vi "Get_parts_list.vi"(7 "LabVIEW Web Service Request":refnum<class "Web Request.lvclass">) -> (2 "Parts_list":cluster{"String":string, "Value":string}[](array[cluster])=[{"String"="Пластина", "Value"="plate.png"}, {"String"="Вал", "Value"="shaft.png"}, {"String"="Ось", "Value"="axis.png"}, {"String"="Диск", "Value"="disk.png"}, {"String"="Кольцо", "Value"="ring.png"}, {"String"="Втулка", "Value"="bushing.png"}, {"String"="Крыльчатка", "Value"="impeller.png"}, {"String"="Лезвийный инструмент", "Value"="blade_tool.png"}])   [LabVIEW 2020]
uses:
  <vilib>/wsapi/Web Request.lvclass
panel:
  # "Use the Web Service Request input terminal to call the VIs on the Web Services palette. Do not remove it from the connector pane unless you don't need access to the palette."
  # "Each additional control wired to the connector pane will be available as an input in the URL. To include an indicator in terminal-mode output (the default setting), it must also be wired to the connector pane."
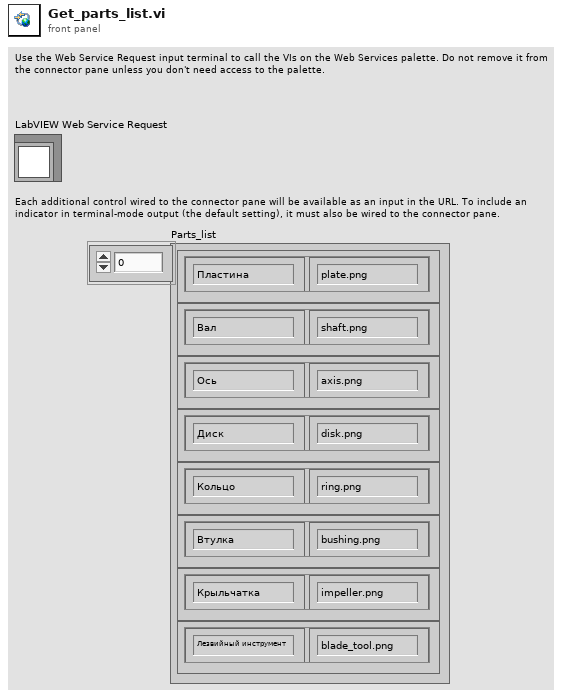
[diagram p1: front panel]
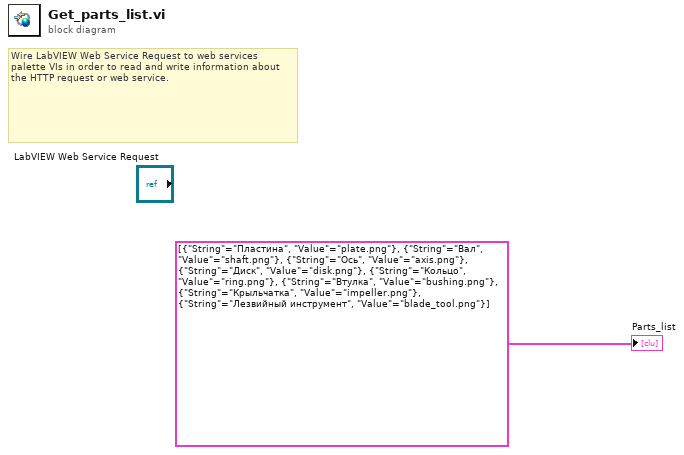
[diagram p0: block diagram]
diagram:
  # "Wire LabVIEW Web Service Request to web services palette VIs in order to read and write information about the HTTP request or web service."
  "Parts_list" <- cluster{"String":string, "Value":string}[] [{"String"="Пластина", "Value"="plate.png"}, {"String"="Вал", "Value"="shaft.png"}, {"String"="Ось", "Value"="axis.png"}, {"String"="Диск", "Value"="disk.png"}, {"String"="Кольцо", "Value"="ring.png"}, {"String"="Втулка", "Value"="bushing.png"}, {"String"="Крыльчатка", "Value"="impeller.png"}, {"String"="Лезвийный инструмент", "Value"="blade_tool.png"}]
